vi "Handle Find DQMH Broadcast Events in vilib.vi"(8 "Action":enum16{"Read", "Write", "Delete"}(ring)) -> (3 "Exist":bool)   [LabVIEW 2020, in "Panther Dashboard.lvlib"]
doc: "The intention of this VI is to\nEnable/Disable Panther Dashboard\nUIS, when Disabled, the Default\nDQMH UIs will be Used"
uses:
  Panther Dashboard.lvlib
  <resource>/dialog/lvconfig.llb/LV Config Read String.vi
  <resource>/dialog/lvconfig.llb/LV Config Write String.vi
panel:
  out "error out":errorcluster
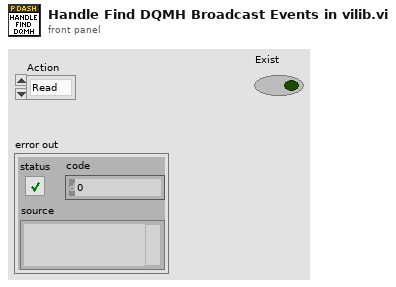
[diagram p1: front panel]
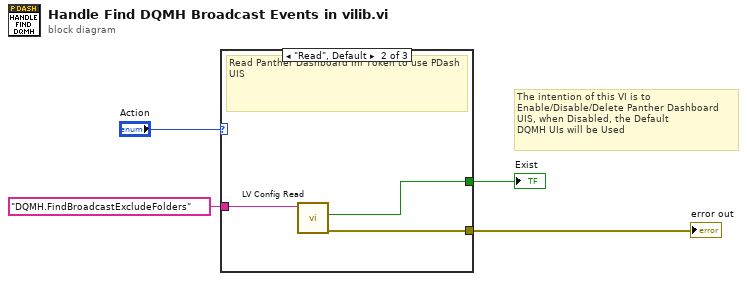
[diagram p0: block diagram]
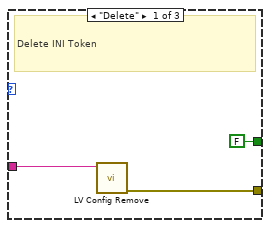
[diagram p2: hidden frame]
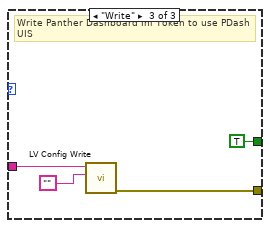
[diagram p3: hidden frame]
diagram:
  # "The intention of this VI is to\nEnable/Disable/Delete Panther Dashboard\nUIS, when Disabled, the Default\nDQMH UIs will be Used"
  n1 = case shown="\"Read\", Default" "Action" {
    tunnel: "DQMH.FindBroadcastExcludeFolders" ("key") -> [w6 w9 w13]
    tunnel: [FALSE ("found?") w8 TRUE ("found?")] -> w2
    tunnel: [w7 w10 w14] -> w4
    frame "Delete" {
      # "Delete INI Token"
      n2 = call <resource>:"LV Config Remove.vi"("key"=w6) -> ("error out"=w7:errorcluster)  [unwired: 6 in]
    }
    frame "Read", Default {
      # "Read Panther Dashboard Ini Token to use PDash UIS"
      n3 = call-poly <resource>:"LV Config Read.vi"("key"=w9) -> ("error out"=w10:errorcluster, "found?"=w8:bool)  [unwired: 4 in, 1 out]
    }
    frame "Write" {
      # "Write Panther Dashboard Ini Token to use PDash UIS"
      n4 = call-poly <resource>:"LV Config Write.vi"("value"="", "key"=w13) -> ("error out"=w14:errorcluster)  [unwired: 5 in]
    }
  }
  "Exist" <- w2
  "error out" <- w4
